vi "TDMS Process.vi"(8 "error in (no error)":errorcluster, 11 "View Model":T1) -> (0 "error out":errorcluster)   [LabVIEW 2017]
doc: "Implementation of TDMS process which responsible for Logging all necessary data to external TDMS files."
uses:
  View Model/Controls/View Model.ctl
  View Model/Controls/Shared Model.ctl
  Error Handler/Controls/Error Model.ctl
  Error Handler/Controls/Error Event.ctl
  Error Handler/Controls/Error Type.ctl
  Controller/Controls/Controller Model.ctl
  Controller/Controls/Controller Event.ctl
  Controller/Controls/Controller Command.ctl
  Controller/Controls/Controller Overhead.ctl
  Real-Time/RT Status.ctl
  Real-Time/RT Loop Status.ctl
  Controller/Controls/Controller NStream.ctl
  Controller/Controls/Controller DAQ Data.ctl
  Controls/TDMS Model.ctl
  Controls/TDMS Event.ctl
  Controls/TDMS Command.ctl
  Controls/TDMS Overhead.ctl
  Controls/TDMS ChanNames.ctl
  Classes/Reports/TDMS/TDMS.lvclass
  D:/Work/LVProjects/CANDU/src/Classes/Reports/Log/Log.lvclass
  Classes/Reports/TDMS/TDMS.lvclass/TDMS.ctl
  Classes/Reports/Log/Log.lvclass/Log.ctl
  Classes/Reports/Log/Log.lvclass
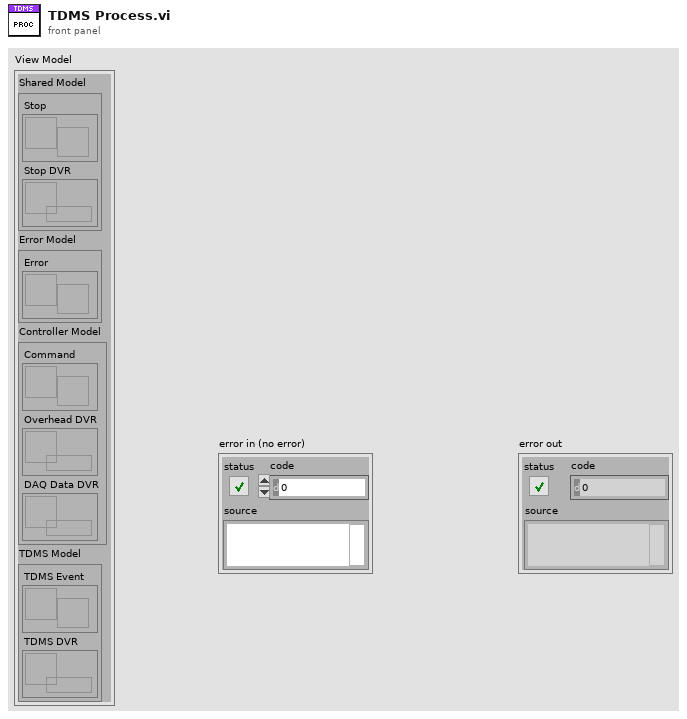
[diagram p1: front panel]
types:
  T1 = typedef "View Model.ctl" = cluster{"Shared Model":T2, "Error Model":T3, "Controller Model":T4, "TDMS Model":T5}
  T2 = typedef "Shared Model.ctl" = cluster{"Stop":refnum<user-event>, "Stop DVR":refnum<data-value>}
  T3 = typedef "Error Model.ctl" = cluster{"Error":refnum<user-event>}
  T4 = typedef "Controller Model.ctl" = cluster{"Command":refnum<user-event>, "Overhead DVR":refnum<data-value>, "DAQ Data DVR":refnum<data-value>}
  T5 = typedef "TDMS Model.ctl" = cluster{"TDMS Event":refnum<user-event>, "TDMS DVR":refnum<data-value>}
  T6 = typedef "Error Type.ctl" = enum16{"Minor", "Critical"}
  T7 = typedef "TDMS Command.ctl" = enum16{"Idle", "Create File", "Save Data", "Close Fire"}
  T8 = typedef "Controller Command.ctl" = enum16{"Idle", "Init", "Stop App", "Stop RT", "NStream Create", "NStream Begin", "NStream End", "NStream Close", "DAQ Data Read", "DAQ Data Write", "TDMS Restart"}
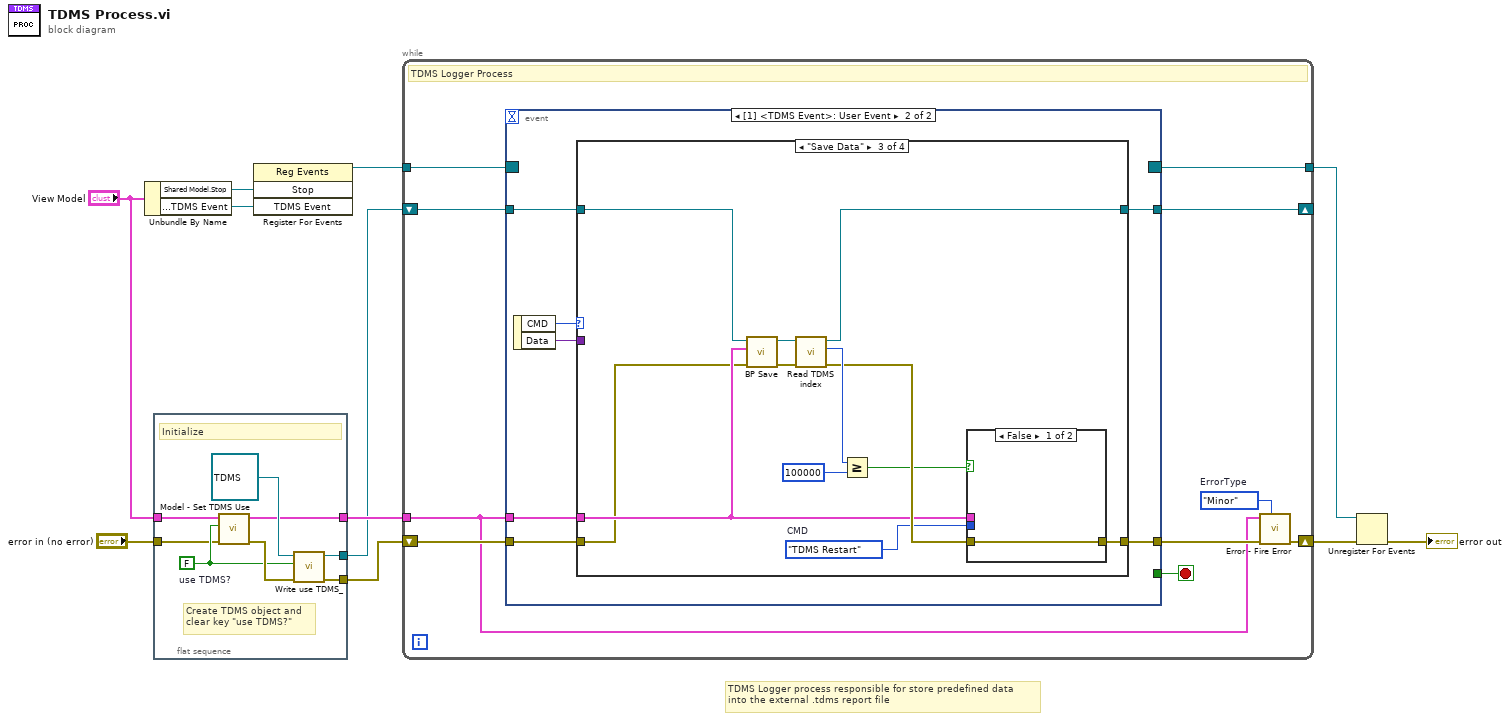
[diagram p0: block diagram]
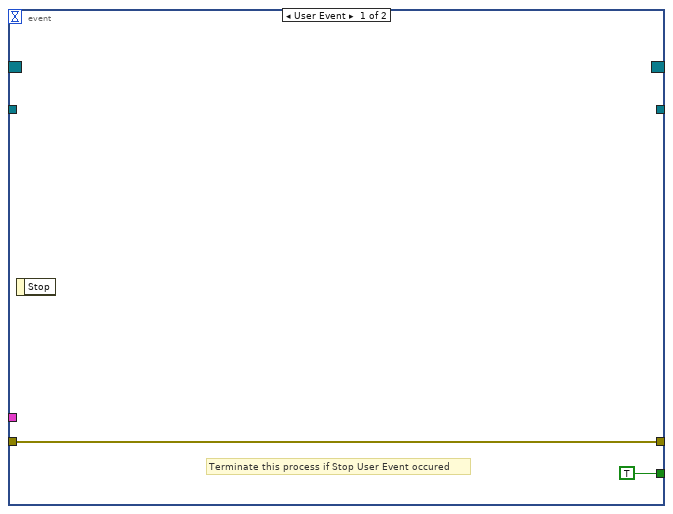
[diagram p2: hidden frame]
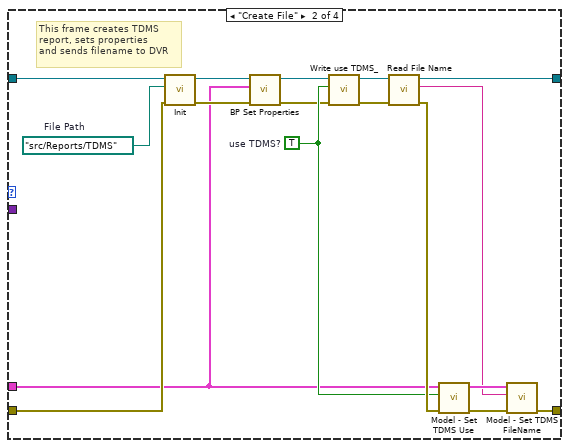
[diagram p4: hidden frame]
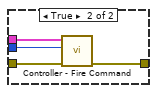
[diagram p5: hidden frame]
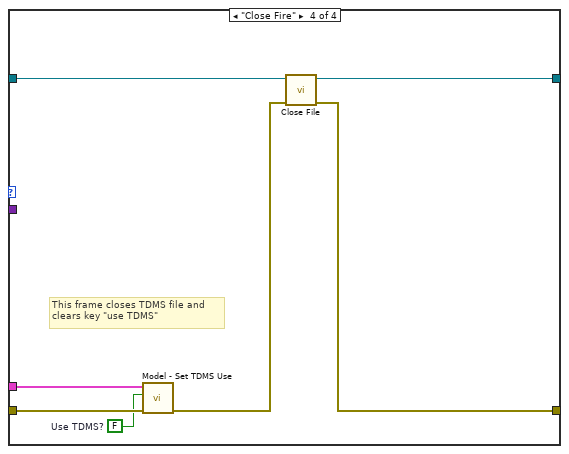
[diagram p6: hidden frame]
diagram:
  # "TDMS Logger process responsible for store predefined data\ninto the external .tdms report file"
  n1 = Unbundle By Name("View Model") -> ("Shared Model.Stop"=w11:refnum<user-event>, "TDMS Model.TDMS Event"=w6:refnum<user-event>)
  n2 = flat-sequence {
    tunnel: "error in (no error)" -> [w16]
    tunnel: "View Model" -> [w15]
    tunnel: [w14] -> w3
    tunnel: [w13] -> w2
    tunnel: [w12] -> w1
    frame #0 {
      w17 = FALSE  # use TDMS?
      # "Create TDMS object and\nclear key \"use TDMS?\""
      # "Initialize"
      n3 = call "Model - Set TDMS Use.vi"("error in (no error)"=w16, "Use TDMS?"=w17, "View Model"=w15) -> ("error out"=w18:errorcluster, "View Model"=w13:T1)  [unwired: 7 in]
      n4 = call "Write use TDMS_.vi"("error in"=w18, "use TDMS?"=w17, "TDMS in"=refnum<class "TDMS.lvclass"> refnum ("Report_lib.lvlib:TDMS.lvclass")) -> ("error out"=w14:errorcluster, "TDMS out"=w12:refnum<class "TDMS.lvclass">)  [unwired: 7 in]
    }
  }
  n5 = register-events(w11, w6) -> (reference out=w10:refnum<event-registration>)  [unwired: 2 in, 1 out]
  n6 = while {
    tunnel: w10 -> [w28]
    shift-right: [w24] -> w9
    shift-left: w3 -> [w29]
    tunnel: w2 -> [w23]
    tunnel: [w27] -> w8
    shift-right: [w21] -> _
    shift-left: w1 -> [w20]
    stop <- w26 stop-if-true
    w22 = Error_Type."Minor"  # ErrorType
    # "TDMS Logger Process"
    n7 = event shown="[1] <TDMS Event>: User Event" {
      selector: w28 -> [_ _]
      dyn-events: [_ _] -> w27
      timeout: _ -> [_ _]
      tunnel: w29 -> [w31 w35]
      tunnel: w23 -> [_ w36]
      tunnel: [w31 w34] -> w25
      tunnel: [TRUE _] -> w26
      tunnel: [_ w33] -> w21
      tunnel: w20 -> [_ w32]
      event User Event {
        # "Terminate this process if Stop User Event occured"
        n8 = event-data() -> ()  [unwired: 1 in, 1 out]
      }
      event User Event {
        n9 = event-data() -> ("CMD"=w38:T7, "Data"=w37:variant)  [unwired: 1 in]
        n10 = case shown="\"Save Data\"" w38 {
          tunnel: w37 -> [_ _ _ _]
          tunnel: w36 -> [_ w41 w59 w80]
          tunnel: w35 -> [w39 w52 w58 w81]
          tunnel: [w39 w55 w65 w75] -> w34
          tunnel: [w40 w47 w67 w77] -> w33
          tunnel: w32 -> [w40 w57 w60 w78]
          frame "Idle", Default {
          }
          frame "Create File" {
            w46 = path "src/Reports/TDMS"  # File Path
            w49 = TRUE  # use TDMS?
            # "This frame creates TDMS\nreport, sets properties\nand sends filename to DVR"
            n11 = call "Init.vi"("error in"=w52, "File Path"=w46, "TDMS in"=w57) -> ("error out"=w44:errorcluster, "TDMS out"=w45:refnum<class "TDMS.lvclass">)  [unwired: 7 in]
            n12 = call "BP Set Properties.vi"("error in"=w44, "View Model in"=w41, "TDMS in"=w45) -> ("error out"=w43:errorcluster, "TDMS out"=w42:refnum<class "TDMS.lvclass">)  [unwired: 7 in]
            n13 = call "Write use TDMS_.vi"("error in"=w43, "use TDMS?"=w49, "TDMS in"=w42) -> ("error out"=w50:errorcluster, "TDMS out"=w53:refnum<class "TDMS.lvclass">)  [unwired: 7 in]
            n14 = call "Read File Name.vi"("error in (no error)"=w50, "Log in"=w53) -> ("error out"=w51:errorcluster, "File Name"=w48:string, "Log out"=w47:refnum<class "TDMS.lvclass">)  [unwired: 7 in]
            n15 = call "Model - Set TDMS Use.vi"("error in (no error)"=w51, "Use TDMS?"=w49, "View Model"=w41) -> ("error out"=w54:errorcluster, "View Model"=w56:T1)  [unwired: 7 in]
            n16 = call "Model - Set TDMS FileName.vi"("error in (no error)"=w54, "FileName"=w48, "View Model"=w56) -> ("error out"=w55:errorcluster)  [unwired: 7 in, 1 out]
          }
          frame "Save Data" {
            w63 = Controller_Command."TDMS Restart"  # CMD
            n17 = call "BP Save.vi"("error in"=w58, "View Model in"=w59, "TDMS in"=w60) -> ("error out"=w61:errorcluster, "TDMS out"=w62:refnum<class "TDMS.lvclass">)  [unwired: 7 in]
            n18 = call "Read TDMS index.vi"("error in"=w61, "TDMS in"=w62) -> ("error out"=w66:errorcluster, "TDMS index"=w69:i32, "TDMS out"=w67:refnum<class "TDMS.lvclass">)  [unwired: 7 in]
            n19 = Greater Or Equal?(x=w69, y=100000) -> (x >= y?=w64:bool)
            n20 = case shown="False" w64 {
              tunnel: w66 -> [w70 w74]
              tunnel: w59 -> [_ w73]
              tunnel: [w70 w72] -> w65
              tunnel: w63 -> [_ w71]
              frame False {
              }
              frame True {
                n21 = call "Controller - Fire Command.vi"("error in (no error)"=w74, "CMD"=w71, "View Model"=w73) -> ("error out"=w72:errorcluster)  [unwired: 8 in]
              }
            }
          }
          frame "Close Fire" {
            w79 = FALSE  # Use TDMS?
            # "This frame closes TDMS file and \nclears key \"use TDMS\""
            n22 = call "Model - Set TDMS Use.vi"("error in (no error)"=w81, "Use TDMS?"=w79, "View Model"=w80) -> ("error out"=w76:errorcluster)  [unwired: 7 in, 1 out]
            n23 = call-dynamic "Close File.vi"("error in"=w76, "TDMS in"=w78) -> ("error out"=w75:errorcluster, "TDMS out"=w77:refnum<class "TDMS.lvclass">)  [unwired: 8 in]
          }
        }
      }
    }
    n24 = call "Error - Fire Error.vi"("ErrorType"=w22, "error in (no error)"=w25, "View Model"=w23) -> ("error out"=w24:errorcluster)  [unwired: 7 in, 1 out]
  }
  n25 = Unregister For Events(event registration refnum=w8, error in=w9) -> (error out=→"error out":errorcluster)
